vi "Begin.vi"(8 "error in":errorcluster) -> (0 "error out":errorcluster)   [LabVIEW 2019]
doc: "Called before other user functions, this VI can be used to open I/O refnums, load in file data, and do general program initialization. Notice that the <B>error out</B> terminal is simply used for data flow. Wiring it to other structures or subVIs ensures that this VI runs first."
uses:
  <vilib>/Rock Robotics/WPI/DriverStation/WPI_DriverStationRobotMode2.ctl
  <vilib>/Rock Robotics/WPI/Joystick/WPI_JoystickDeviceEnum.ctl
  <vilib>/Rock Robotics/SystemInterfaces/DIO/FPGA_DIOPWMChannel.ctl
  <vilib>/Rock Robotics/WPI/SafetyOutput/WPI_SafetyOutputConfigMenu.ctl
  Robot Global Data.vi
  <vilib>/Rock Robotics/WPI/RobotDrive/WPI_RobotDriveOpen2MotorWithExistingMotors.vi
  <vilib>/Rock Robotics/WPI/MotorControl/WPI_MotorControlOpen SPARK.vi
  <vilib>/Rock Robotics/Network Tables/NT Write String Array.vi
  <vilib>/Rock Robotics/WPI/Solenoid/WPI_SolenoidOpenSingle.vi
  <vilib>/Rock Robotics/WPI/Solenoid/WPI_SolenoidSetEnum.vi
  <vilib>/Rock Robotics/WPI/Solenoid/WPI_SolenoidChannel.ctl
  <vilib>/Rock Robotics/WPI/Solenoid/WPI_SolenoidValue.ctl
  <vilib>/Rock Robotics/Network Tables/NT Write Boolean Array.vi
  <vilib>/Rock Robotics/Network Tables/NT Write Numeric Array.vi
panel:
  in  "Calibration Time (sec)":u32=4
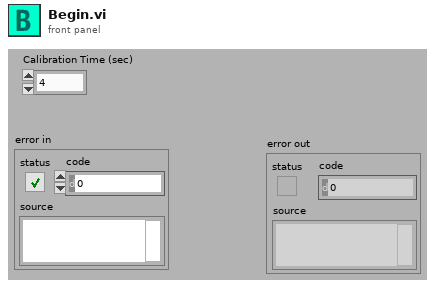
[diagram p1: front panel]
types:
  T1 = typedef "WPI_SafetyOutputConfigMenu.ctl" = enum16{"Enable", "Disable"}
  T2 = typedef "FPGA_DIOPWMChannel.ctl" = enum8{"PWM 0", "PWM 1", "PWM 2", "PWM 3", "PWM 4", "PWM 5", "PWM 6", "PWM 7", "PWM 8", "PWM 9", "PWM MXP 0", "PWM MXP 1", "PWM MXP 2", "PWM MXP 3", "PWM MXP 4", "PWM MXP 5", "PWM MXP 6", "PWM MXP 7", "PWM MXP 8", "PWM MXP 9", "Invalid"}
  T3 = typedef "WPI_JoystickDeviceEnum.ctl" = enum16{"USB 0", "USB 1", "USB 2", "USB 3", "USB 4", "USB 5"}
  T4 = typedef "WPI_DriverStationRobotMode2.ctl" = enum16{"Autonomous Disabled", "Autonomous Enabled", "Teleop Disabled", "Teleop Enabled", "Disconnected", "Finish", "Test Disabled", "Test Enabled", "Emergency Stopped"}
  T5 = typedef "WPI_JoystickDevRef.ctl" = cluster{"Device":T3}
  T6 = typedef "WPI_MotorControlDeviceRef.ctl" = cluster{"DeviceStatus":errorcluster, "Type":T7, "PWM":cluster{"PWM Channel":T2, "DeadBand":T8}, "CAN":cluster{"Device Number":u8, "SetOutput VI Ref":variant, "GetOutput VI Ref":variant, "Enable VI Ref":variant, "Disable VI Ref":variant, "Data":variant}, "Invert":bool, "DIO PWM":cluster{"PWM \"Enable\" Channel":T2, "DIOChannel":T9, "PWM Rate":dbl}}
  T7 = typedef "WPI_MotorControlType.ctl" = enum16{"PWM", "CAN", "DIO PWM"}
  T8 = typedef "WPI_PWMDeadband.ctl" = cluster{"Name":string, "maxPositivePwm":i32, "minPositivePwm":i32, "centerPwm":i32, "maxNegativePwm":i32, "minNegativePwm":i32, "angularRange":u16}
  T9 = typedef "FPGA_DIOChannel.ctl" = enum8{"DIO 0", "DIO 1", "DIO 2", "DIO 3", "DIO 4", "DIO 5", "DIO 6", "DIO 7", "DIO 8", "DIO 9", "DIO MXP 0", "DIO MXP 1", "DIO MXP 2", "DIO MXP 3", "DIO MXP 4", "DIO MXP 5", "DIO MXP 6", "DIO MXP 7", "DIO MXP 8", "DIO MXP 9", "DIO MXP 10", "DIO MXP 11", "DIO MXP 12", "DIO MXP 13", "DIO MXP 14", "DIO MXP 15", "SPI Port CS1", "SPI Port CS2", "SPI Port CS3", "SPI Port MISO", "SPI Port MOSI", "Invalid"}
  T10 = typedef "WPI_RobotDriveDevRef.ctl" = cluster{"DevStatus":errorcluster, "Motors[]":T6[], "Square Inputs":bool, "Max Output":dbl}
  T11 = typedef "ADIS 16448 HW Configuration.ctl" = cluster{"SPI Clock Rate (Hz)":dbl, "IMU SPI Mode (3)":T12, "IMU Reset Pin":T9, "IMU SPI Bus":T13, "IMU Data Ready Pin":T9, "Stall Config":cluster{"Pow2BytesPerRead":u8, "StallTicks":u16, "CsToSclkTicks":u8}, "IMU Status LED Pin":T9}
  T12 = typedef "WPI_SPIMode.ctl" = enum16{"Mode 0 (Clk Idle Low,Sample on Leading)", "Mode 1 (Clk Idle Low,Sample on Trailing)", "Mode 2 (Clk Idle High,Sample on Leading)", "Mode 3 (Clk Idle High,Sample on Trailing)"}
  T13 = typedef "spi_bus.ctl" = enum16{"SPI On-Board, CS0", "SPI On-Board, CS1", "SPI On-Board, CS2", "SPI On-Board, CS3", "SPI MXP", "Invalid"}
  T14 = typedef "WPI_SolenoidValue.ctl" = enum16{"Off", "On", "Forward", "Reverse"}
  T15 = typedef "WPI_SolenoidChannel.ctl" = enum8{"Solenoid 0", "Solenoid 1", "Solenoid 2", "Solenoid 3", "Solenoid 4", "Solenoid 5", "Solenoid 6", "Solenoid 7", "Invalid"}
  T16 = typedef "WPI_SolenoidDevRef.ctl" = cluster{"DevStatus":errorcluster, "Pneumatics Control Module":u8, "Forward Solenoid Channel":T15, "Reverse Solenoid Channel":T15}
  T17 = typedef "ADIS16448 Device Reference.ctl" = cluster{"DevStatus":errorcluster, "Hardware Config":T18, "Calibration Complete":refnum<notifier>, "Status FIFO":refnum<k33>, "Last Value Reference":refnum<data-value>, "Sychronous Process VI":T19, "Cmd FIFO":refnum<k33>, "Source":T20, "Data FIFO":refnum<k33>, "IMU Status LED Pin":T9, "Calibration Time":u32}
  T18 = typedef "ADIS16448 Hardware Configuration.ctl" = cluster{"SPI Clock Rate (Hz)":dbl, "IMU SPI Mode (3)":T12, "IMU Reset Pin":T9, "IMU SPI Bus":T13, "IMU Data Ready Pin":T9, "Stall Config":cluster{"Pow2BytesPerRead":u8, "StallTicks":u16, "CsToSclkTicks":u8}, "IMU Status LED Pin":T9}
  T19 = typedef "ADIS16448 Process.ctl" = refnum<vi>
  T20 = typedef "FPGA_CounterEncoderSourceConvertionLVSourceType.ctl" = cluster{"DevStatus":errorcluster, "AnalogTriggerMode?":bool, "DigitalMode":cluster{"DIO Channel":T21}, "AnalogTriggerMode":cluster{"AnalogTriggerIndex":T22, "OutputType":T23}}
  T21 = typedef "FPGA_DIODigitalSourceChannel.ctl" = enum8{"DIO 0", "DIO 1", "DIO 2", "DIO 3", "DIO 4", "DIO 5", "DIO 6", "DIO 7", "DIO 8", "DIO 9", "DIO MXP 0", "DIO MXP 1", "DIO MXP 2", "DIO MXP 3", "DIO MXP 4", "DIO MXP 5", "DIO MXP 6", "DIO MXP 7", "DIO MXP 8", "DIO MXP 9", "DIO MXP 10", "DIO MXP 11", "DIO MXP 12", "DIO MXP 13", "DIO MXP 14", "DIO MXP 15", "SPI Port CS1", "SPI Port CS2", "SPI Port CS3", "SPI Port MISO", "SPI Port MOSI", "Disabled"}
  T22 = typedef "FPGA_AnalogTriggerIndex.ctl" = enum8{"Trig 0", "Trig 1", "Trig 2", "Trig 3", "Trig 4", "Trig 5", "Trig 6", "Trig 7", "Invalid"}
  T23 = typedef "FPGA_AnalogTriggerOutType.ctl" = enum16{"InWindow", "TriggerState", "Rising", "Falling"}
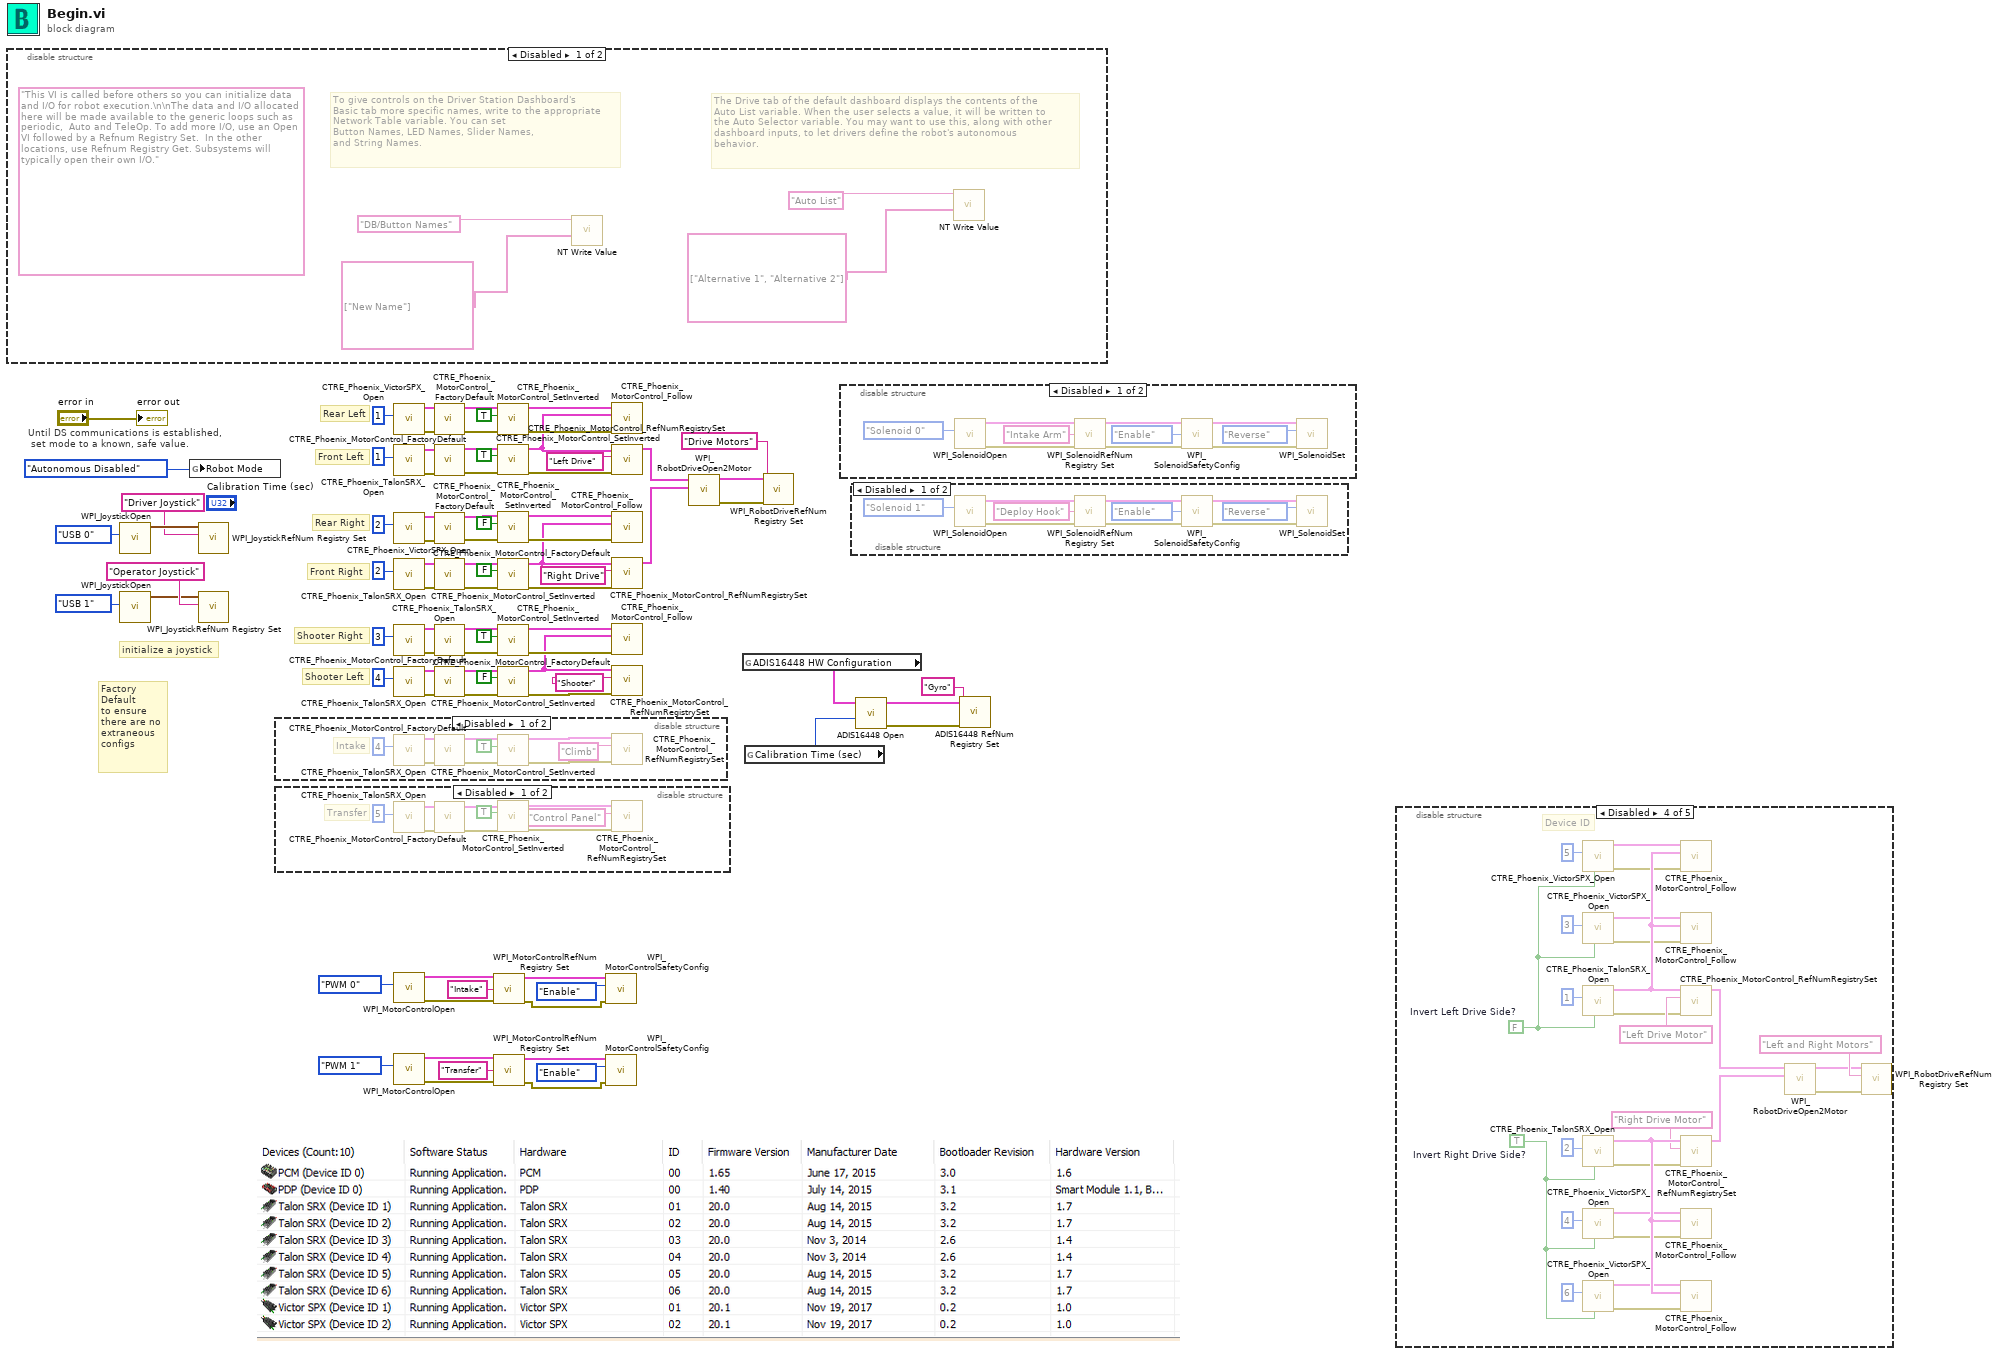
[diagram p0: block diagram]
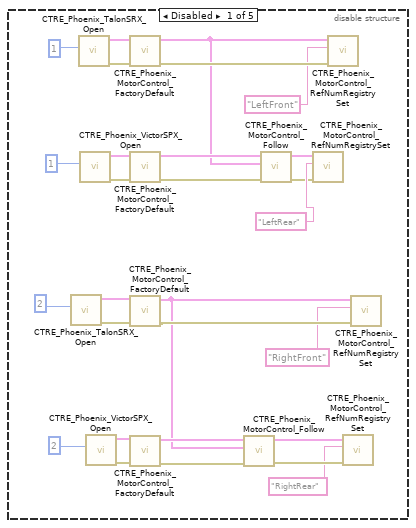
[diagram p6: hidden frame]
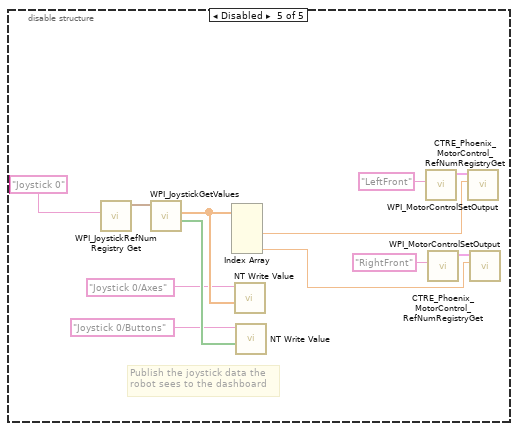
[diagram p9: hidden frame]
diagram:
  # "Shooter Left"
  # "Shooter Right"
  # "Factory \nDefault \nto ensure \nthere are no \nextraneous \nconfigs"
  # "Front Right"
  # "Front Left"
  # "Rear Right"
  # "Rear Left"
  # "initialize a joystick"
  # "Until DS communications is established,\n set mode to a known, safe value."
  n1 = disable-structure shown="Disabled" {
    frame Disabled {
      (unwired) "This VI is called before others so you can initialize data and I/O for robot execution.\n\nThe data and I/O allocated here will be made available to the generic loops such as periodic,  Auto and TeleOp. To add more I/O, use an Open VI followed by a Refnum Registry Set.  In the other locations, use Refnum Registry Get. Subsystems will typically open their own I/O."
      # "The Drive tab of the default dashboard displays the contents of the\nAuto List variable. When the user selects a value, it will be written to\nthe Auto Selector variable. You may want to use this, along with other\ndashboard inputs, to let drivers define the robot's autonomous\nbehavior."
      # "To give controls on the Driver Station Dashboard's\nBasic tab more specific names, write to the appropriate\nNetwork Table variable. You can set\nButton Names, LED Names, Slider Names,\nand String Names."
      n2 = call-poly <vilib>:"NT Write Value.vi"("String Array"=string[] ["New Name"], "Name"="DB/Button Names") -> ()  [unwired: 9 in, 1 out]
      n3 = call-poly <vilib>:"NT Write Value.vi"("String Array"=string[] ["Alternative 1", "Alternative 2"], "Name"="Auto List") -> ()  [unwired: 9 in, 1 out]
    }
    frame Enabled {
    }
  }
  n4 = call <vilib>:"WPI_JoystickOpen.vi"("JoystickDevice"=WPI_JoystickDeviceEnum."USB 0") -> ("JoystickDevRef"=w66:T5)  [unwired: 10 in]
  n5 = call <vilib>:"WPI_JoystickOpen.vi"("JoystickDevice"=WPI_JoystickDeviceEnum."USB 1") -> ("JoystickDevRef"=w81:T5)  [unwired: 10 in]
  n6 = global write "Robot Global Data.vi" "Robot Mode"(WPI_DriverStationRobotMode2."Autonomous Disabled" ("Robot Mode")) -> ()
  n7 = call <vilib>:"WPI_JoystickRefNum Registry Set.vi"("refnum name"="Driver Joystick", "JoystickDevRef"=w66) -> ()  [unwired: 8 in, 2 out]
  n8 = call <vilib>:"WPI_JoystickRefNum Registry Set.vi"("refnum name"="Operator Joystick", "JoystickDevRef"=w81) -> ()  [unwired: 8 in, 2 out]
  n9 = disable-structure shown="Disabled" {
    frame Disabled {
      # "Intake"
      n10 = call <vilib>:"CTRE_Phoenix_TalonSRX_Open.vi"("Device Number"=u8 4) -> ("error out"=w94:errorcluster, "CAN Talon SRX Ref"=w93:T6)  [unwired: 9 in]
      n11 = call <vilib>:"CTRE_Phoenix_MotorControl_FactoryDefault.vi"("error in"=w94, "PhoenixMotorControlDevRef"=w93) -> ("error out"=w90:errorcluster, "PhoenixMotorControlDevRef"=w91:T6)  [unwired: 8 in]
      n12 = call <vilib>:"CTRE_Phoenix_MotorControl_SetInverted.vi"("error in (no error)"=w90, "Invert?"=TRUE, "PhoenixMotorControlDevRef"=w91) -> ("error out"=w89:errorcluster, "PhoenixMotorControlDevRef"=w88:T6)  [unwired: 7 in]
      n13 = call <vilib>:"CTRE_Phoenix_MotorControl_RefNumRegistrySet.vi"("error in (no error)"=w89, "refnum name"="Climb", "PhoenixMotorControlDevRef"=w88) -> ()  [unwired: 7 in, 2 out]
    }
    frame Enabled {
    }
  }
  n14 = disable-structure shown="Disabled" {
    frame Disabled {
      # "Transfer"
      n15 = call <vilib>:"CTRE_Phoenix_TalonSRX_Open.vi"("Device Number"=u8 5) -> ("error out"=w103:errorcluster, "CAN Talon SRX Ref"=w102:T6)  [unwired: 9 in]
      n16 = call <vilib>:"CTRE_Phoenix_MotorControl_FactoryDefault.vi"("error in"=w103, "PhoenixMotorControlDevRef"=w102) -> ("error out"=w99:errorcluster, "PhoenixMotorControlDevRef"=w100:T6)  [unwired: 8 in]
      n17 = call <vilib>:"CTRE_Phoenix_MotorControl_SetInverted.vi"("error in (no error)"=w99, "Invert?"=TRUE, "PhoenixMotorControlDevRef"=w100) -> ("error out"=w98:errorcluster, "PhoenixMotorControlDevRef"=w97:T6)  [unwired: 7 in]
      n18 = call <vilib>:"CTRE_Phoenix_MotorControl_RefNumRegistrySet.vi"("error in (no error)"=w98, "refnum name"="Control Panel", "PhoenixMotorControlDevRef"=w97) -> ()  [unwired: 7 in, 2 out]
    }
    frame Enabled {
    }
  }
  n19 = call <vilib>:"CTRE_Phoenix_VictorSPX_Open.vi"("Device Number"=u8 1) -> ("error out"=w64:errorcluster, "CAN Talon SRX Ref"=w63:T6)  [unwired: 9 in]
  n20 = call <vilib>:"CTRE_Phoenix_TalonSRX_Open.vi"("Device Number"=u8 1) -> ("error out"=w61:errorcluster, "CAN Talon SRX Ref"=w62:T6)  [unwired: 9 in]
  n21 = call <vilib>:"CTRE_Phoenix_VictorSPX_Open.vi"("Device Number"=u8 2) -> ("error out"=w60:errorcluster, "CAN Talon SRX Ref"=w59:T6)  [unwired: 9 in]
  n22 = call <vilib>:"CTRE_Phoenix_TalonSRX_Open.vi"("Device Number"=u8 2) -> ("error out"=w58:errorcluster, "CAN Talon SRX Ref"=w57:T6)  [unwired: 9 in]
  n23 = call <vilib>:"CTRE_Phoenix_TalonSRX_Open.vi"("Device Number"=u8 3) -> ("error out"=w19:errorcluster, "CAN Talon SRX Ref"=w18:T6)  [unwired: 9 in]
  n24 = call <vilib>:"CTRE_Phoenix_TalonSRX_Open.vi"("Device Number"=u8 4) -> ("error out"=w17:errorcluster, "CAN Talon SRX Ref"=w16:T6)  [unwired: 9 in]
  n25 = call-poly <vilib>:"WPI_MotorControlOpen.vi"("PWM Channel"=FPGA_DIOPWMChannel."PWM 0") -> ("error out"=w31:errorcluster, "MotorControlDeviceRef"=w35:T6)  [unwired: 9 in]
  n26 = call-poly <vilib>:"WPI_MotorControlOpen.vi"("PWM Channel"=FPGA_DIOPWMChannel."PWM 1") -> ("error out"=w28:errorcluster, "MotorControlDeviceRef"=w24:T6)  [unwired: 9 in]
  n27 = call <vilib>:"CTRE_Phoenix_MotorControl_FactoryDefault.vi"("error in"=w64, "PhoenixMotorControlDevRef"=w63) -> ("error out"=w55:errorcluster, "PhoenixMotorControlDevRef"=w54:T6)  [unwired: 8 in]
  n28 = call <vilib>:"CTRE_Phoenix_MotorControl_FactoryDefault.vi"("error in"=w61, "PhoenixMotorControlDevRef"=w62) -> ("error out"=w49:errorcluster, "PhoenixMotorControlDevRef"=w50:T6)  [unwired: 8 in]
  n29 = call <vilib>:"CTRE_Phoenix_MotorControl_FactoryDefault.vi"("error in"=w60, "PhoenixMotorControlDevRef"=w59) -> ("error out"=w45:errorcluster, "PhoenixMotorControlDevRef"=w44:T6)  [unwired: 8 in]
  n30 = call <vilib>:"CTRE_Phoenix_MotorControl_FactoryDefault.vi"("error in"=w58, "PhoenixMotorControlDevRef"=w57) -> ("error out"=w40:errorcluster, "PhoenixMotorControlDevRef"=w39:T6)  [unwired: 8 in]
  n31 = call <vilib>:"CTRE_Phoenix_MotorControl_FactoryDefault.vi"("error in"=w19, "PhoenixMotorControlDevRef"=w18) -> ("error out"=w13:errorcluster, "PhoenixMotorControlDevRef"=w14:T6)  [unwired: 8 in]
  n32 = call <vilib>:"CTRE_Phoenix_MotorControl_FactoryDefault.vi"("error in"=w17, "PhoenixMotorControlDevRef"=w16) -> ("error out"=w8:errorcluster, "PhoenixMotorControlDevRef"=w9:T6)  [unwired: 8 in]
  n33 = call <vilib>:"WPI_MotorControlRefNum Registry Set.vi"("error in (no error)"=w31, "refnum name"="Intake", "MotorControlDevRef"=w35) -> ("error out"=w30:errorcluster, "MotorControlDevRef"=w34:T6)  [unwired: 7 in]
  n34 = call <vilib>:"WPI_MotorControlRefNum Registry Set.vi"("error in (no error)"=w28, "refnum name"="Transfer", "MotorControlDevRef"=w24) -> ("error out"=w29:errorcluster, "MotorControlDevRef"=w25:T6)  [unwired: 7 in]
  n35 = call <vilib>:"CTRE_Phoenix_MotorControl_SetInverted.vi"("error in (no error)"=w55, "Invert?"=TRUE, "PhoenixMotorControlDevRef"=w54) -> ("error out"=w52:errorcluster, "PhoenixMotorControlDevRef"=w53:T6)  [unwired: 7 in]
  n36 = call <vilib>:"CTRE_Phoenix_MotorControl_SetInverted.vi"("error in (no error)"=w49, "Invert?"=TRUE, "PhoenixMotorControlDevRef"=w50) -> ("error out"=w48:errorcluster, "PhoenixMotorControlDevRef"=w47:T6)  [unwired: 7 in]
  n37 = call <vilib>:"CTRE_Phoenix_MotorControl_SetInverted.vi"("error in (no error)"=w45, "Invert?"=FALSE, "PhoenixMotorControlDevRef"=w44) -> ("error out"=w42:errorcluster, "PhoenixMotorControlDevRef"=w43:T6)  [unwired: 7 in]
  n38 = call <vilib>:"CTRE_Phoenix_MotorControl_SetInverted.vi"("error in (no error)"=w40, "Invert?"=FALSE, "PhoenixMotorControlDevRef"=w39) -> ("error out"=w37:errorcluster, "PhoenixMotorControlDevRef"=w38:T6)  [unwired: 7 in]
  n39 = call <vilib>:"CTRE_Phoenix_MotorControl_SetInverted.vi"("error in (no error)"=w13, "Invert?"=TRUE, "PhoenixMotorControlDevRef"=w14) -> ("error out"=w12:errorcluster, "PhoenixMotorControlDevRef"=w11:T6)  [unwired: 7 in]
  n40 = call <vilib>:"CTRE_Phoenix_MotorControl_SetInverted.vi"("error in (no error)"=w8, "Invert?"=FALSE, "PhoenixMotorControlDevRef"=w9) -> ("error out"=w7:errorcluster, "PhoenixMotorControlDevRef"=w6:T6)  [unwired: 7 in]
  n41 = call <vilib>:"WPI_MotorControlSafetyConfig.vi"("error in (no error)"=w30, "mode"=WPI_SafetyOutputConfigMenu."Enable", "MotorControlDevRef"=w34) -> ()  [unwired: 7 in, 2 out]
  n42 = call <vilib>:"WPI_MotorControlSafetyConfig.vi"("error in (no error)"=w29, "mode"=WPI_SafetyOutputConfigMenu."Enable", "MotorControlDevRef"=w25) -> ()  [unwired: 7 in, 2 out]
  n43 = call <vilib>:"CTRE_Phoenix_MotorControl_Follow.vi"("error in (no error)"=w52, "Master Controller to Follow"=w47, "PhoenixMotorControlDevRef"=w53) -> ()  [unwired: 7 in, 2 out]
  n44 = call <vilib>:"CTRE_Phoenix_MotorControl_RefNumRegistrySet.vi"("error in (no error)"=w48, "refnum name"="Left Drive", "PhoenixMotorControlDevRef"=w47) -> ("PhoenixMotorControlDevRef"=w74:T6)  [unwired: 7 in, 1 out]
  n45 = call <vilib>:"CTRE_Phoenix_MotorControl_Follow.vi"("error in (no error)"=w42, "Master Controller to Follow"=w38, "PhoenixMotorControlDevRef"=w43) -> ()  [unwired: 7 in, 2 out]
  n46 = call <vilib>:"CTRE_Phoenix_MotorControl_RefNumRegistrySet.vi"("error in (no error)"=w37, "refnum name"="Right Drive", "PhoenixMotorControlDevRef"=w38) -> ("PhoenixMotorControlDevRef"=w73:T6)  [unwired: 7 in, 1 out]
  n47 = call <vilib>:"CTRE_Phoenix_MotorControl_Follow.vi"("error in (no error)"=w12, "Master Controller to Follow"=w6, "PhoenixMotorControlDevRef"=w11) -> ()  [unwired: 7 in, 2 out]
  n48 = call <vilib>:"CTRE_Phoenix_MotorControl_RefNumRegistrySet.vi"("error in (no error)"=w7, "refnum name"="Shooter", "PhoenixMotorControlDevRef"=w6) -> ()  [unwired: 7 in, 2 out]
  n49 = call-poly <vilib>:"WPI_RobotDriveOpen2Motor.vi"("Right Motor Dev Ref"=w73, "Left Motor Dev Ref"=w74) -> ("error out"=w69:errorcluster, "RobotDriveDevRef"=w70:T10)  [unwired: 8 in]
  n50 = global read "Robot Global Data.vi" "ADIS16448 HW Configuration"() -> (w5:T11)
  n51 = global read "Robot Global Data.vi" "Calibration Time (sec)"() -> (w4:u32)
  n52 = call <vilib>:"WPI_RobotDriveRefNum Registry Set.vi"("error in (no error)"=w69, "refnum name"="Drive Motors", "RobotDriveDevRef"=w70) -> ()  [unwired: 7 in, 2 out]
  n53 = disable-structure shown="Disabled" {
    frame Disabled {
      n54 = call-poly <vilib>:"WPI_SolenoidOpen.vi"("Solenoid Channel"=WPI_SolenoidChannel."Solenoid 0") -> ("error out"=w112:errorcluster, "SolenoidDevRef"=w115:T16)  [unwired: 9 in]
      n55 = call <vilib>:"WPI_SolenoidRefNum Registry Set.vi"("error in (no error)"=w112, "refnum name"="Intake Arm", "SolenoidDevRef"=w115) -> ("error out"=w111:errorcluster, "SolenoidDevRef"=w114:T16)  [unwired: 7 in]
      n56 = call <vilib>:"WPI_SolenoidSafetyConfig.vi"("error in (no error)"=w111, "mode"=WPI_SafetyOutputConfigMenu."Enable", "SolenoidDevRef"=w114) -> ("error out"=w110:errorcluster, "SolenoidDevRef"=w113:T16)  [unwired: 7 in]
      n57 = call-poly <vilib>:"WPI_SolenoidSet.vi"("error in (no error)"=w110, "Value"=WPI_SolenoidValue."Reverse", "SolenoidDevRef"=w113) -> ()  [unwired: 7 in, 2 out]
    }
    frame Enabled {
    }
  }
  n58 = disable-structure shown="Disabled" {
    frame Disabled {
      n59 = call-poly <vilib>:"WPI_SolenoidOpen.vi"("Solenoid Channel"=WPI_SolenoidChannel."Solenoid 1") -> ("error out"=w119:errorcluster, "SolenoidDevRef"=w116:T16)  [unwired: 9 in]
      n60 = call <vilib>:"WPI_SolenoidRefNum Registry Set.vi"("error in (no error)"=w119, "refnum name"="Deploy Hook", "SolenoidDevRef"=w116) -> ("error out"=w120:errorcluster, "SolenoidDevRef"=w117:T16)  [unwired: 7 in]
      n61 = call <vilib>:"WPI_SolenoidSafetyConfig.vi"("error in (no error)"=w120, "mode"=WPI_SafetyOutputConfigMenu."Enable", "SolenoidDevRef"=w117) -> ("error out"=w121:errorcluster, "SolenoidDevRef"=w118:T16)  [unwired: 7 in]
      n62 = call-poly <vilib>:"WPI_SolenoidSet.vi"("error in (no error)"=w121, "Value"=WPI_SolenoidValue."Reverse", "SolenoidDevRef"=w118) -> ()  [unwired: 7 in, 2 out]
    }
    frame Enabled {
    }
  }
  n63 = call <vilib>:"ADIS16448 Open.vi"("Initial Calibration Time (sec)"=w4, "Hardware Config"=w5) -> ("error out"=w2:errorcluster, "ADIS16448DevRef"=w3:T17)  [unwired: 8 in]
  n64 = call <vilib>:"ADIS16448 RefNum Registry Set.vi"("error in (no error)"=w2, "refnum name"="Gyro", "ADIS16448DevRef"=w3) -> ()  [unwired: 7 in, 2 out]
  n65 = disable-structure shown="Disabled" {
    frame Disabled {
      n66 = call <vilib>:"CTRE_Phoenix_TalonSRX_Open.vi"("Device Number"=u8 2) -> ("error out"=w150:errorcluster, "CAN Talon SRX Ref"=w140:T6)  [unwired: 9 in]
      n67 = call <vilib>:"CTRE_Phoenix_TalonSRX_Open.vi"("Device Number"=u8 1) -> ("error out"=w148:errorcluster, "CAN Talon SRX Ref"=w138:T6)  [unwired: 9 in]
      n68 = call <vilib>:"CTRE_Phoenix_VictorSPX_Open.vi"("Device Number"=u8 1) -> ("error out"=w146:errorcluster, "CAN Talon SRX Ref"=w144:T6)  [unwired: 9 in]
      n69 = call <vilib>:"CTRE_Phoenix_VictorSPX_Open.vi"("Device Number"=u8 2) -> ("error out"=w152:errorcluster, "CAN Talon SRX Ref"=w142:T6)  [unwired: 9 in]
      n70 = call <vilib>:"CTRE_Phoenix_MotorControl_FactoryDefault.vi"("error in"=w148, "PhoenixMotorControlDevRef"=w138) -> ("error out"=w149:errorcluster, "PhoenixMotorControlDevRef"=w139:T6)  [unwired: 8 in]
      n71 = call <vilib>:"CTRE_Phoenix_MotorControl_FactoryDefault.vi"("error in"=w146, "PhoenixMotorControlDevRef"=w144) -> ("error out"=w147:errorcluster, "PhoenixMotorControlDevRef"=w145:T6)  [unwired: 8 in]
      n72 = call <vilib>:"CTRE_Phoenix_MotorControl_FactoryDefault.vi"("error in"=w150, "PhoenixMotorControlDevRef"=w140) -> ("error out"=w151:errorcluster, "PhoenixMotorControlDevRef"=w141:T6)  [unwired: 8 in]
      n73 = call <vilib>:"CTRE_Phoenix_MotorControl_FactoryDefault.vi"("error in"=w152, "PhoenixMotorControlDevRef"=w142) -> ("error out"=w153:errorcluster, "PhoenixMotorControlDevRef"=w143:T6)  [unwired: 8 in]
      n74 = call <vilib>:"CTRE_Phoenix_MotorControl_Follow.vi"("error in (no error)"=w153, "Master Controller to Follow"=w141, "PhoenixMotorControlDevRef"=w143) -> ("error out"=w136:errorcluster, "PhoenixMotorControlDevRef"=w137:T6)  [unwired: 7 in]
      n75 = call <vilib>:"CTRE_Phoenix_MotorControl_Follow.vi"("error in (no error)"=w147, "Master Controller to Follow"=w139, "PhoenixMotorControlDevRef"=w145) -> ("error out"=w128:errorcluster, "PhoenixMotorControlDevRef"=w129:T6)  [unwired: 7 in]
      n76 = call <vilib>:"CTRE_Phoenix_MotorControl_RefNumRegistrySet.vi"("error in (no error)"=w128, "refnum name"="LeftRear", "PhoenixMotorControlDevRef"=w129) -> ()  [unwired: 7 in, 2 out]
      n77 = call <vilib>:"CTRE_Phoenix_MotorControl_RefNumRegistrySet.vi"("error in (no error)"=w149, "refnum name"="LeftFront", "PhoenixMotorControlDevRef"=w139) -> ()  [unwired: 7 in, 2 out]
      n78 = call <vilib>:"CTRE_Phoenix_MotorControl_RefNumRegistrySet.vi"("error in (no error)"=w136, "refnum name"="RightRear", "PhoenixMotorControlDevRef"=w137) -> ()  [unwired: 7 in, 2 out]
      n79 = call <vilib>:"CTRE_Phoenix_MotorControl_RefNumRegistrySet.vi"("error in (no error)"=w151, "refnum name"="RightFront", "PhoenixMotorControlDevRef"=w141) -> ()  [unwired: 7 in, 2 out]
    }
    frame Enabled {
    }
    frame Disabled {
    }
    frame Disabled {
      w180 = FALSE  # Invert Left Drive Side?
      w179 = TRUE  # Invert Right Drive Side?
      # "Device ID"
      n80 = call <vilib>:"CTRE_Phoenix_VictorSPX_Open.vi"("Invert"=w180, "Device Number"=u8 5) -> ("error out"=w170:errorcluster, "CAN Talon SRX Ref"=w171:T6)  [unwired: 8 in]
      n81 = call <vilib>:"CTRE_Phoenix_VictorSPX_Open.vi"("Invert"=w180, "Device Number"=u8 3) -> ("error out"=w169:errorcluster, "CAN Talon SRX Ref"=w172:T6)  [unwired: 8 in]
      n82 = call <vilib>:"CTRE_Phoenix_TalonSRX_Open.vi"("Invert"=w180, "Device Number"=u8 1) -> ("error out"=w160:errorcluster, "CAN Talon SRX Ref"=w173:T6)  [unwired: 8 in]
      n83 = call <vilib>:"CTRE_Phoenix_TalonSRX_Open.vi"("Invert"=w179, "Device Number"=u8 2) -> ("error out"=w161:errorcluster, "CAN Talon SRX Ref"=w168:T6)  [unwired: 8 in]
      n84 = call <vilib>:"CTRE_Phoenix_VictorSPX_Open.vi"("Invert"=w179, "Device Number"=u8 4) -> ("error out"=w164:errorcluster, "CAN Talon SRX Ref"=w165:T6)  [unwired: 8 in]
      n85 = call <vilib>:"CTRE_Phoenix_VictorSPX_Open.vi"("Invert"=w179, "Device Number"=u8 6) -> ("error out"=w167:errorcluster, "CAN Talon SRX Ref"=w166:T6)  [unwired: 8 in]
      n86 = call <vilib>:"CTRE_Phoenix_MotorControl_Follow.vi"("error in (no error)"=w170, "Master Controller to Follow"=w173, "PhoenixMotorControlDevRef"=w171) -> ()  [unwired: 7 in, 2 out]
      n87 = call <vilib>:"CTRE_Phoenix_MotorControl_Follow.vi"("error in (no error)"=w169, "Master Controller to Follow"=w173, "PhoenixMotorControlDevRef"=w172) -> ()  [unwired: 7 in, 2 out]
      n88 = call <vilib>:"CTRE_Phoenix_MotorControl_RefNumRegistrySet.vi"("error in (no error)"=w160, "refnum name"="Left Drive Motor", "PhoenixMotorControlDevRef"=w173) -> ("PhoenixMotorControlDevRef"=w174:T6)  [unwired: 7 in, 1 out]
      n89 = call <vilib>:"CTRE_Phoenix_MotorControl_RefNumRegistrySet.vi"("error in (no error)"=w161, "refnum name"="Right Drive Motor", "PhoenixMotorControlDevRef"=w168) -> ("PhoenixMotorControlDevRef"=w175:T6)  [unwired: 7 in, 1 out]
      n90 = call <vilib>:"CTRE_Phoenix_MotorControl_Follow.vi"("error in (no error)"=w164, "Master Controller to Follow"=w168, "PhoenixMotorControlDevRef"=w165) -> ()  [unwired: 7 in, 2 out]
      n91 = call <vilib>:"CTRE_Phoenix_MotorControl_Follow.vi"("error in (no error)"=w167, "Master Controller to Follow"=w168, "PhoenixMotorControlDevRef"=w166) -> ()  [unwired: 7 in, 2 out]
      n92 = call-poly <vilib>:"WPI_RobotDriveOpen2Motor.vi"("Right Motor Dev Ref"=w175, "Left Motor Dev Ref"=w174) -> ("error out"=w176:errorcluster, "RobotDriveDevRef"=w177:T10)  [unwired: 8 in]
      n93 = call <vilib>:"WPI_RobotDriveRefNum Registry Set.vi"("error in (no error)"=w176, "refnum name"="Left and Right Motors", "RobotDriveDevRef"=w177) -> ()  [unwired: 7 in, 2 out]
    }
    frame Disabled {
      # "Publish the joystick data the\nrobot sees to the dashboard"
      n94 = call <vilib>:"WPI_JoystickRefNum Registry Get.vi"("refnum name"="Joystick 0") -> ("JoystickDevRef"=w182:T5)  [unwired: 1 in, 9 out]
      n95 = call <vilib>:"WPI_JoystickGetValues.vi"("JoystickDevRef"=w182) -> ("Buttons"=w186:bool[], "Axes"=w185:dbl[])  [unwired: 6 in, 3 out]
      n96 = Index Array(array=w185) -> (element #2=w189:dbl, element #4=w192:dbl)  [unwired: 4 in, 2 out]
      n97 = call-poly <vilib>:"NT Write Value.vi"("Numeric Array"=w185, "Name"="Joystick 0/Axes") -> ()  [unwired: 9 in, 1 out]
      n98 = call-poly <vilib>:"NT Write Value.vi"("Boolean Array"=w186, "Name"="Joystick 0/Buttons") -> ()  [unwired: 9 in, 1 out]
      n99 = call <vilib>:"CTRE_Phoenix_MotorControl_RefNumRegistryGet.vi"("refnum name"="LeftFront") -> ("PhoenixMotorControlDevRef"=w188:T6)  [unwired: 9 in, 1 out]
      n100 = call <vilib>:"CTRE_Phoenix_MotorControl_RefNumRegistryGet.vi"("refnum name"="RightFront") -> ("PhoenixMotorControlDevRef"=w191:T6)  [unwired: 9 in, 1 out]
      n101 = call <vilib>:"WPI_MotorControlSetOutput.vi"("Output"=w189, "MotorControlDevRef"=w188) -> ()  [unwired: 7 in, 3 out]
      n102 = call <vilib>:"WPI_MotorControlSetOutput.vi"("Output"=w192, "MotorControlDevRef"=w191) -> ()  [unwired: 7 in, 3 out]
    }
  }
  "error out" <- "error in"
